vi "DBVar TriggeredByData.vi"(1 "data classification":T1(ring), 2 "type  classification":T2(ring), 3 "Not Equal to GenData?":bool) -> (0 "Trigger?":bool)   [LabVIEW 2017, in "NI_DB Variant To Data Support.lvlib"]
uses:
  <vilib>/addons/database/_DB Variant To Data/NI_DB Variant To Data Support.lvlib
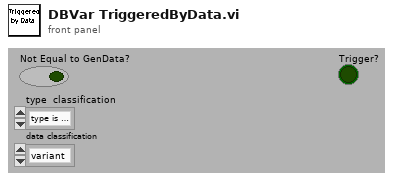
[diagram p1: front panel]
types:
  T1 = enum16{"variant", "variant 1D array", "variant 2D array", "others"}
  T2 = enum16{"type is cluster", "type is 1D array of scalar type", "type is 1D array of cluster type", "type is 2D array", "type is others", "type is unwired"}
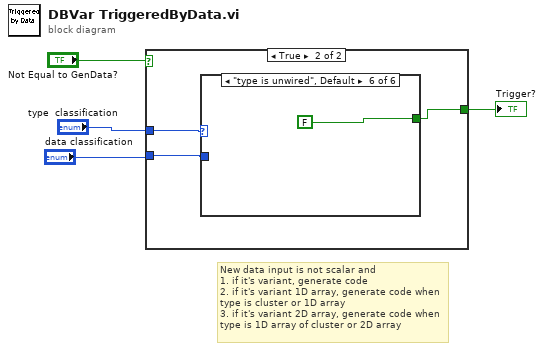
[diagram p0: block diagram]
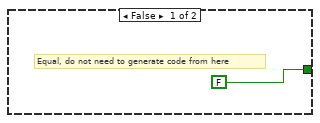
[diagram p2: hidden frame]
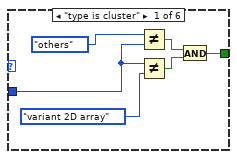
[diagram p3: hidden frame]
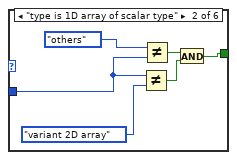
[diagram p4: hidden frame]
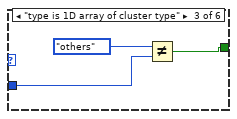
[diagram p5: hidden frame]
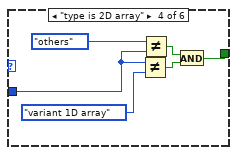
[diagram p6: hidden frame]
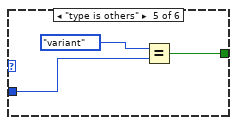
[diagram p7: hidden frame]
diagram:
  # "New data input is not scalar and \n1. if it's variant, generate code\n2. if it's variant 1D array, generate code when type is cluster or 1D array\n3. if it's variant 2D array, generate code when type is 1D array of cluster or 2D array"
  n1 = case shown="True" "Not Equal to GenData?" {
    tunnel: "data classification" -> [_ w7]
    tunnel: [FALSE w6] -> w1
    tunnel: "type  classification" -> [_ w8]
    frame False {
      # "Equal, do not need to generate code from here"
    }
    frame True {
      n2 = case shown="\"type is unwired\", Default" w8 {
        tunnel: w7 -> [w10 w20 w23 w29 w32 _]
        tunnel: [w9 w15 w21 w24 w30 FALSE] -> w6
        frame "type is cluster" {
          n3 = Not Equal?(x=T1."others" ("GenData"), y=w10) -> (x != y?=w12:bool)
          n4 = Not Equal?(x=w10, y=T1."variant 2D array" ("GenData")) -> (x != y?=w11:bool)
          n5 = And(x=w12, y=w11) -> (x .and. y?=w9:bool)
        }
        frame "type is 1D array of scalar type" {
          n6 = Not Equal?(x=w20, y=T1."variant 2D array" ("GenData")) -> (x != y?=w16:bool)
          n7 = Not Equal?(x=T1."others" ("GenData"), y=w20) -> (x != y?=w17:bool)
          n8 = And(x=w17, y=w16) -> (x .and. y?=w15:bool)
        }
        frame "type is 1D array of cluster type" {
          n9 = Not Equal?(x=T1."others" ("GenData"), y=w23) -> (x != y?=w21:bool)
        }
        frame "type is 2D array" {
          n10 = Not Equal?(x=w29, y=T1."variant 1D array" ("GenData")) -> (x != y?=w25:bool)
          n11 = Not Equal?(x=T1."others" ("GenData"), y=w29) -> (x != y?=w26:bool)
          n12 = And(x=w26, y=w25) -> (x .and. y?=w24:bool)
        }
        frame "type is others" {
          n13 = Equal?(x=T1."variant" ("GenData"), y=w32) -> (x = y?=w30:bool)
        }
        frame "type is unwired", Default {
        }
      }
    }
  }
  "Trigger?" <- w1
